vi "Cryo-Con Set Loop Type.vi"(6 "Change control state":bool, 8 "error in (no error)":errorcluster, 9 "Loop number":i32=1, 10 "Set T":T1=enum."Manual", 11 "VISA Resource Name":refnum<visa-resource-name>) -> (0 "error out":errorcluster, 3 "VISA Resource Name Out":refnum<visa-resource-name>)   [LabVIEW 2021]
uses:
  Temperature Controller/Controls/Control Mode.ctl
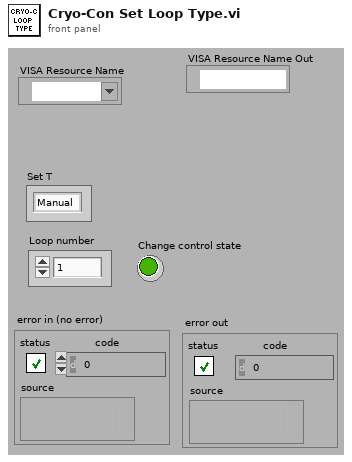
[diagram p1: front panel]
types:
  T1 = typedef "Control Mode.ctl" = enum16{"Off", "PID", "Ramp", "Manual", "Table"}
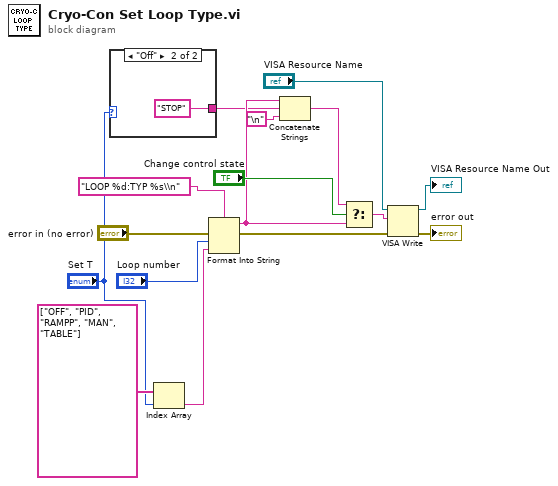
[diagram p0: block diagram]
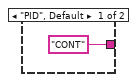
[diagram p2: hidden frame]
diagram:
  n1 = case shown="\"Off\"" "Set T" {
    tunnel: ["CONT" "STOP"] -> w4
    frame "PID", Default {
    }
    frame "Off" {
    }
  }
  n2 = Index Array(array=string[] ["OFF", "PID", "RAMPP", "MAN", "TABLE"] ("string array"), index="Set T") -> (element=w9:string)
  n3 = Format Into String(format string="LOOP %d:TYP %s\\n", error in="error in (no error)", "Loop number", w9) -> (resulting string=w5:string, error out=w15:errorcluster)  [unwired: 1 in]
  n4 = Concatenate Strings(w5, w4, "\n") -> (w2:string)
  n5 = Select(t=w2, s="Change control state", f=w5) -> (s? t:f=w1:string)
  n6 = VISA Write(VISA resource name="VISA Resource Name", write buffer=w1, error in (no error)=w15) -> (VISA resource name out=→"VISA Resource Name Out":refnum<visa-resource-name>, error out=→"error out":errorcluster)  [unwired: 1 out]
